vi "字符串替换.vi"() -> ()   [LabVIEW 2018]
panel:
  out "结果字符串":string
  in  "字符串":string
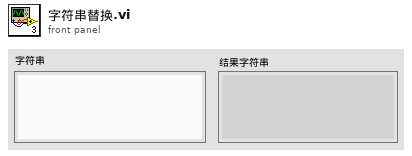
[diagram p1: front panel]
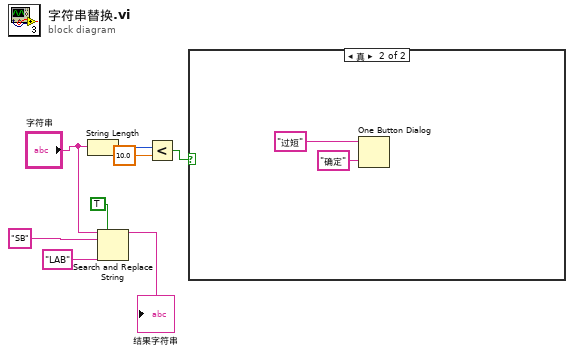
[diagram p0: block diagram]
diagram:
  n1 = String Length(string="字符串") -> (length=w7:i32)
  n2 = Search and Replace String(replace all?=TRUE ("替换全部？(F)"), input string="字符串", search string="SB" ("搜索字符串"), replace string="LAB" ("替换字符串(\"\")")) -> (result string=→"结果字符串":string)  [unwired: 4 in, 3 out]
  n3 = Less?(x=w7, y=10.0) -> (x < y?=w6:bool)
  n4 = case shown="真" w6 {
    frame False {
    }
    frame True {
      n5 = One Button Dialog(message="过短", button name ("OK")="确定" ("按钮名称（“确定”）")) -> ()  [unwired: 1 out]
    }
  }
